vi "Close CAN Device.vi"(8 "error in (no error)":errorcluster, 11 "Cluster in":refnum<vi>) -> (0 "error out":errorcluster, 3 "Return Val":T1=1 items=["OK"=1, "ERROR1"=0, "ERROR2"=-1])   [LabVIEW 2017]
uses:
  PCAN_Driver/ControlCAN.llb/Return Val.ctl
  PCAN_Driver/ControlCAN.lvlib
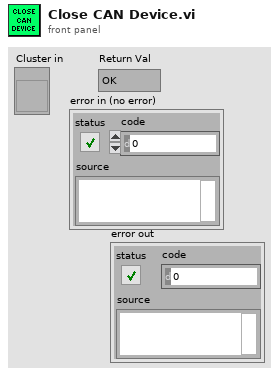
[diagram p1: front panel]
types:
  T1 = typedef "ControlCAN.lvlib/Return Val.ctl" = i32
  T2 = typedef "ControlCAN.lvlib/DevType.ctl" = u32
  T3 = typedef "ControlCAN.lvlib/CAN Channel.ctl" = u32
  T4 = typedef "ControlCAN.lvlib/VCI_INIT_CONFIG.ctl" = cluster{"AccCode":u32, "AccMask":u32, "InitFlag":T5, "Fliter":T6, "Timing0":u8, "Timing1":u8, "Mode":T7}
  T5 = typedef "ControlCAN.lvlib/InitFlag.ctl" = u32
  T6 = typedef "ControlCAN.lvlib/Fliter.ctl" = u8
  T7 = typedef "ControlCAN.lvlib/Mode.ctl" = u8
  T8 = cluster{"DevType":T2, "DevIndex":u32, "CanIndex":T3, "VCI_INIT_CONFIG":T4}
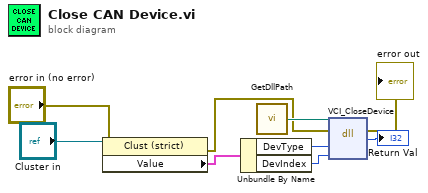
[diagram p0: block diagram]
diagram:
  n1 = property class="Clust (strict)"(reference="Cluster in", error in="error in (no error)") -> (error out=w2:errorcluster, "Value"=w7:T8)  [unwired: 1 out]
  n2 = Unbundle By Name(w7) -> ("DevType"=w6:T2, "DevIndex"=w5:u32)
  n3 = call "GetDllPath.vi"() -> ("DllPath"=w9:path)  [unwired: 1 in]
  n4 = dll-call lib="C:/Projects/Marvin CAN UTD/MarvinATP/data/ControlCAN.dll" fn="VCI_CloseDevice"(path in=w9, error in=w2, "DevType"=w6, "DevIndex"=w5) -> (error out=→"error out":errorcluster, "ReturnVal"=→"Return Val":i32)  [unwired: 3 in, 1 out]
